vi "未命名 3.vi"(0 "A":dbl, 1 "B":dbl) -> (2 "A+B":dbl, 3 "布尔":bool, 4 "A*B":dbl)   [LabVIEW 2012]
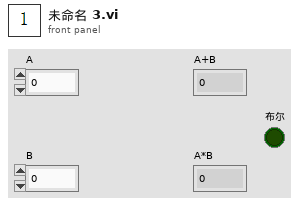
[diagram p1: front panel]
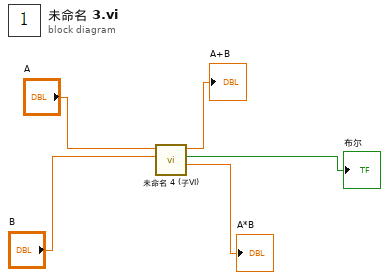
[diagram p0: block diagram]
diagram:
  n1 = call "未命名 4 (子VI).vi"("B"="B", "A"="A") -> ("A*B"=→"A*B":dbl, "布尔"=→"布尔":bool, "A+B"=→"A+B":dbl)  [unwired: 7 in]
